vi "hCtlParams.vi"(6 "hID":string, 7 "LabVIEW Web Service Request":refnum<class "Web Request.lvclass">, 9 "D":dbl, 10 "I":dbl, 11 "P":dbl) -> ()   [LabVIEW 2014]
uses:
  <vilib>/wsapi/Web Request.lvclass
  Controller/Controller.lvclass
  reusable/Session APIs/CVT/CVT.lvclass
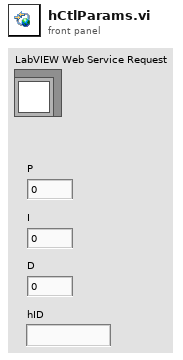
[diagram p1: front panel]
types:
  T1 = typedef "Session - Root.lvclass/Session Handle.ctl" = refnum<data-value>
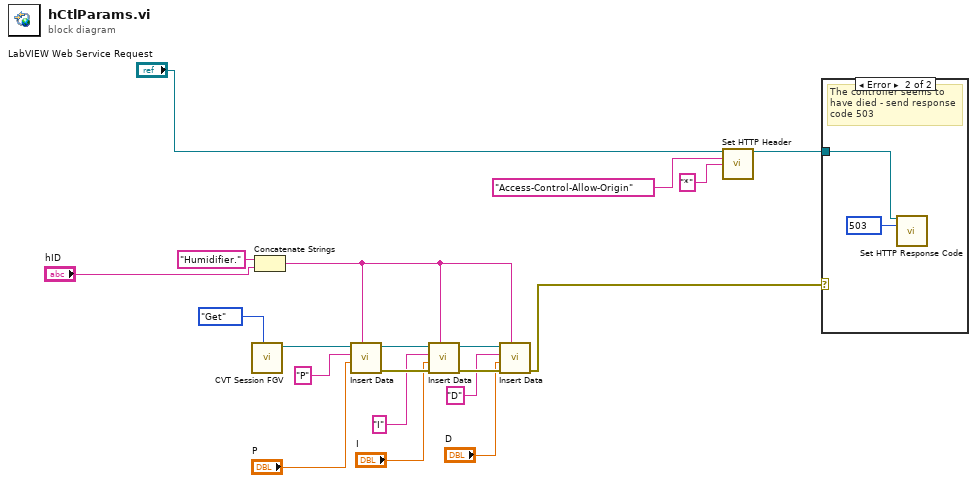
[diagram p0: block diagram]
diagram:
  n1 = call "CVT Session FGV.vi"("State"=enum16{"Init", "Get"}."Get") -> ("CVT Session Out"=w15:T1)  [unwired: 10 in]
  n2 = Concatenate Strings("Humidifier." ("string"), "hID") -> (w3:string)
  n3 = call "Insert Data.vi"("Group"=w3, "Data"="P", "tag"="P", "CVT Session In"=w15) -> ("error out"=w8:errorcluster, "CVT Session Out"=w12:T1)  [unwired: 6 in]
  n4 = call "Insert Data.vi"("Group"=w3, "error in"=w8, "Data"="I", "tag"="I", "CVT Session In"=w12) -> ("error out"=w7:errorcluster, "CVT Session Out"=w11:T1)  [unwired: 5 in]
  n5 = call "Insert Data.vi"("Group"=w3, "error in"=w7, "Data"="D", "tag"="D", "CVT Session In"=w11) -> ("error out"=w1:errorcluster)  [unwired: 5 in, 1 out]
  n6 = call <vilib>:"Set HTTP Header.vi"("LabVIEW Web Service Request"="LabVIEW Web Service Request", "header"="Access-Control-Allow-Origin", "header value"="*") -> ("LabVIEW Web Service Request out"=w17:refnum<class "Web Request.lvclass">)  [unwired: 11 in, 1 out]
  n7 = case shown="Error" w1 {
    tunnel: w17 -> [_ w21]
    frame No Error {
    }
    frame Error {
      w22 = 503 items=["100"=100, "101"=101, "200"=200, "201"=201, "202"=202, "203"=203, "204"=204, "205"=205, "206"=206, "300"=300, "301"=301, "302"=302, "303"=303, "304"=304, "305"=305, "306"=306, "307"=307, "400"=400, "401"=401, "402"=402, "403"=403, "404"=404, "405"=405, "406"=406, "407"=407, "408"=408, "409"=409, "410"=410, "411"=411, "412"=412, "413"=413, "414"=414, "415"=415, "416"=416, "417"=417, "500"=500, "501"=501, "502"=502, "503"=503, "504"=504, "505"=505] ("response code (200)")
      # "The controller seems to have died - send response code 503"
      n8 = call <vilib>:"Set HTTP Response Code.vi"("LabVIEW Web Service Request"=w21, "response code (200)"=w22) -> ()  [unwired: 12 in, 2 out]
    }
  }
